vi "hwOperation_Config Signals.vi"(7 "hwType":string, 8 "error in":errorcluster, 10 "Devs Info in":T1[](array[typedef]), 11 "hwDriverRef in":T3) -> (0 "error out":errorcluster, 3 "hwDriverRef out":T3)   [LabVIEW 2016]
uses:
  QX/hw_QX_hwDriverRef.ctl
  C:/Users/CL/Desktop/ZcDAQprj0811/ZcDAQprj/Modules/DAQ-Device/Hardware Drivers/QX/HBM LabVIEW Driver/DLLs/Hbm.Api.Common.dll
  QX/HBM LabVIEW Driver/DLLs/Hbm.Api.Common.dll
  DAQ-Config/Controls/PSCHN_Card Para.ctl
  DAQ-Config/Controls/PSCHN_Channel Para.ctl
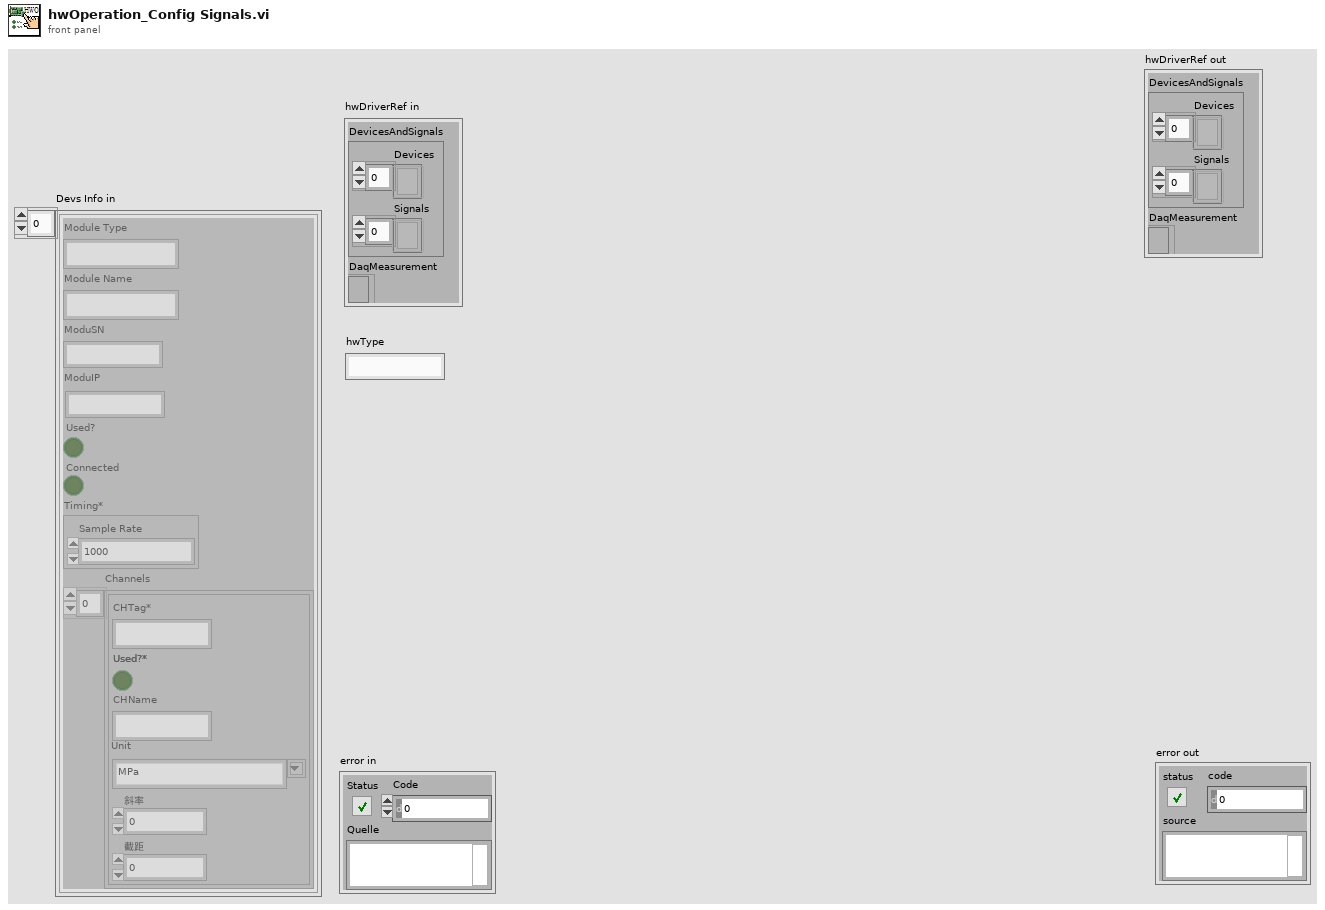
[diagram p1: front panel]
types:
  T1 = typedef "PSCHN_Card Para.ctl" = cluster{"Module Type":string, "Module Name":string, "ModuSN":string, "ModuIP":string, "Used?":bool, "Connected":bool, "Timing*":cluster{"Sample Rate":dbl}, "Channels":T2[]}
  T2 = typedef "PSCHN_Channel Para.ctl" = cluster{"CHTag*":string, "Used?*":bool, "CHName":string, "Unit":string, "斜率":dbl, "截距":dbl}
  T3 = typedef "hw_QX_hwDriverRef.ctl" = cluster{"DevicesAndSignals":cluster{"Devices":refnum<k24>[], "Signals":refnum<k24>[]}, "DaqMeasurement":refnum<k24>}
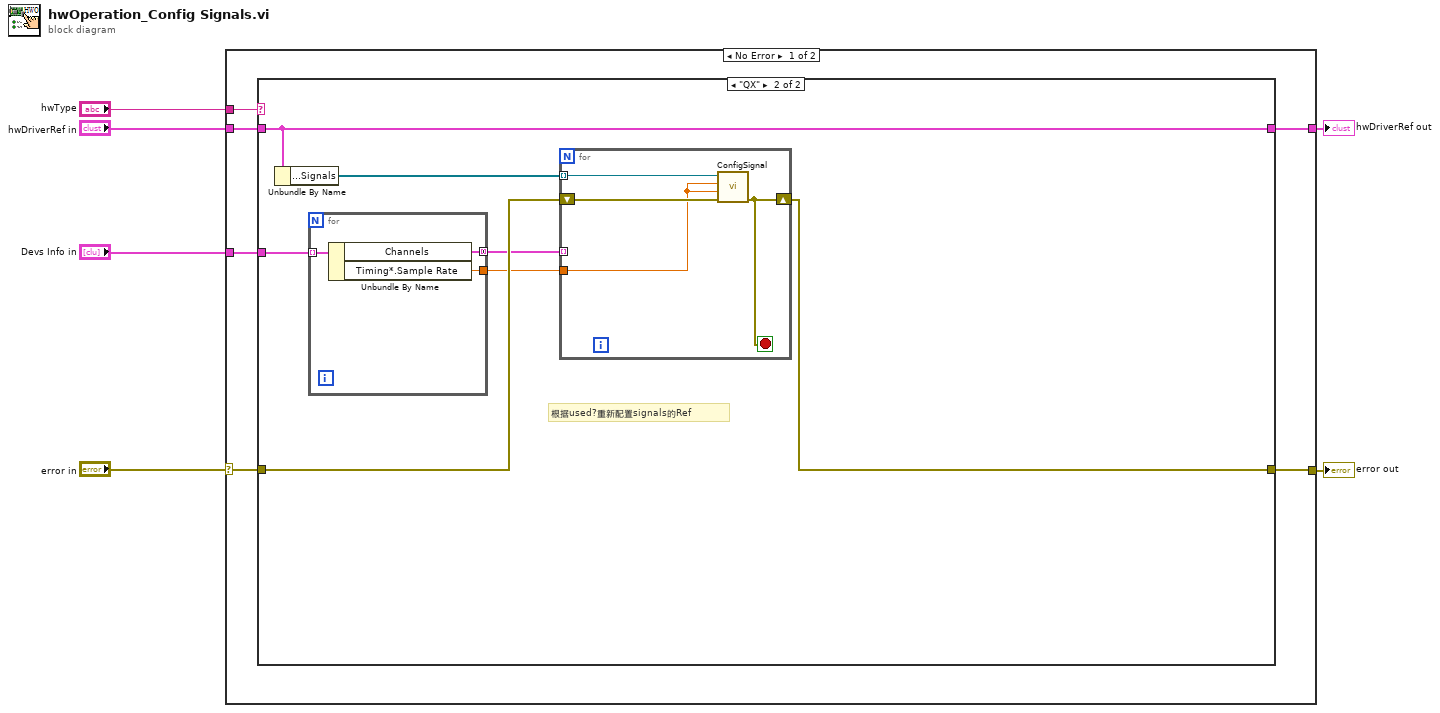
[diagram p0: block diagram]
diagram:
  n1 = case shown="No Error" "error in" {
    selector: "error in" -> [w11 w30]
    tunnel: [w12 w30] -> w5
    tunnel: "hwType" -> [w10 _]
    tunnel: "hwDriverRef in" -> [w9 w29]
    tunnel: [w8 w29] -> w2
    tunnel: "Devs Info in" -> [w7 _]
    frame No Error {
      n2 = case shown="\"QX\"" w10 {
        tunnel: [w14 w20] -> w12
        tunnel: w11 -> [w14 w21]
        tunnel: w9 -> [w13 w16]
        tunnel: [w13 w16] -> w8
        tunnel: w7 -> [_ w19]
        frame "Simulation", Default {
        }
        frame "QX" {
          # "根据used?重新配置signals的Ref"
          n3 = Unbundle By Name(w16) -> ("DevicesAndSignals.Signals"=w17:refnum<k24>[])
          n4 = for {
            tunnel: w19 -> [w24] mode=indexing
            tunnel: [w23] -> w18 mode=concatenating
            tunnel: [w22] -> w15
            n5 = Unbundle By Name(w24) -> ("Channels"=w23:T2[], "Timing*.Sample Rate"=w22:dbl)
          }
          n6 = for {
            tunnel: w17 -> [w27] mode=indexing
            shift-right: [w28] -> w20
            shift-left: w21 -> [w26]
            tunnel: w18 -> [_] mode=indexing
            tunnel: w15 -> [w25]
            stop <- w28 stop-if-true
            n7 = call "ConfigSignal.vi"("Error in"=w26, "SampleRate"=w25, "FilterFrequency"=w25, "Signal"=w27) -> ("Error out"=w28:errorcluster)  [unwired: 7 in]
          }
        }
      }
    }
    frame Error {
    }
  }
  "error out" <- w5
  "hwDriverRef out" <- w2
